vi "generate random numbers.vi"(7 "random seed":dbl, 8 "error in (no error)":errorcluster, 9 "lowlim":dbl, 10 "highlim":dbl=1.0, 11 "number of elements":dbl=10.0) -> (0 "error out":errorcluster, 3 "random numbers":dbl[](array[numeric]))   [LabVIEW 2011]
doc: "Generates user specified number of random numbers, within the limits specified by high and low. The random number seed is provided as a user input, if it is left at the default of zero then the seed is not used."
uses:
  <userlib>/_OpenG.lib/numeric/numeric.llb/Random Number Within Range - DBL__ogtk.vi
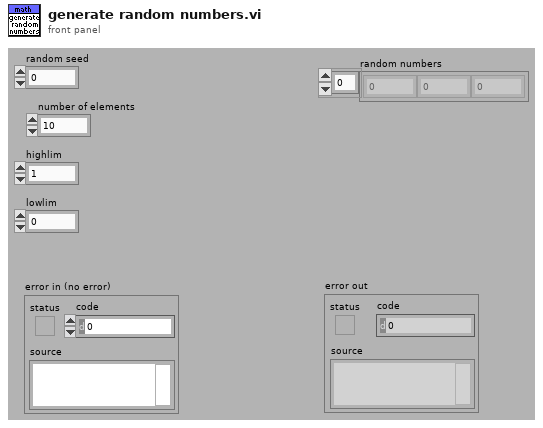
[diagram p1: front panel]
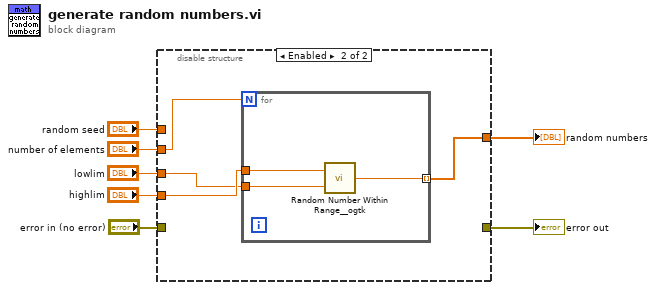
[diagram p0: block diagram]
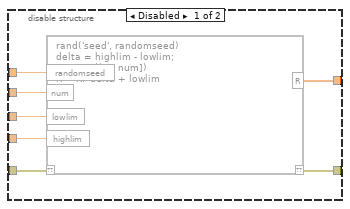
[diagram p2: hidden frame]
diagram:
  n1 = disable-structure shown="Enabled" {
    disable-tunnel: "random seed" -> [w14 _]
    disable-tunnel: "number of elements" -> [w13 w16]
    disable-tunnel: "lowlim" -> [w12 w17]
    disable-tunnel: "highlim" -> [w11 w18]
    disable-tunnel: [w10 w15] -> w3
    disable-tunnel: "error in (no error)" -> [w9 _]
    disable-tunnel: [w8 _] -> w1
    frame Disabled {
      n2 = mathscript code="rand('seed', randomseed)\ndelta = highlim - lowlim;\nR = rand([1, num])\nR = R.*delta + lowlim"("??"=w9, "randomseed"=w14, "num"=w13, "lowlim"=w12, "highlim"=w11) -> ("??"=w8:errorcluster, "R"=w10:dbl[])
    }
    frame Enabled {
      n3 = for {
        N: w16 -> [_]
        tunnel: w18 -> [w21]
        tunnel: w17 -> [w20]
        tunnel: [w19] -> w15 mode=indexing
        n4 = call-poly <userlib>:"Random Number Within Range__ogtk.vi"("High"=w21, "Low"=w20) -> ("Random Number"=w19:dbl)  [unwired: 3 in]
      }
    }
  }
  "random numbers" <- w3
  "error out" <- w1
